vi "sendNoAckToClient.vi"(8 "error in (no error)":errorcluster, 10 "tcpPacket":string, 11 "tcpServerCmd in":refnum<class "TcpServerCmd.lvclass">) -> (0 "error out":errorcluster, 2 "tcpPacket":string, 3 "tcpServerCmd out":refnum<class "TcpServerCmd.lvclass">)   [LabVIEW 2018, in "TcpServerCmd.lvclass"]
doc: "Send the noAck to the TCP Client."
uses:
  TcpServerCmd.lvclass
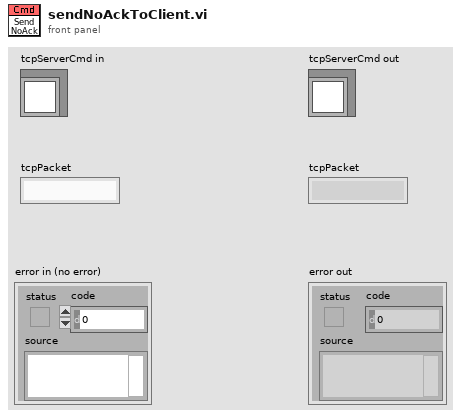
[diagram p1: front panel]
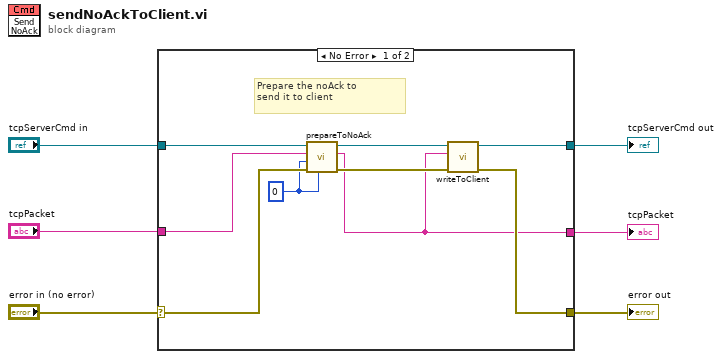
[diagram p0: block diagram]
diagram:
  n1 = case shown="No Error" "error in (no error)" {
    selector: "error in (no error)" -> [w11 w18]
    tunnel: [w14 w18] -> w5
    tunnel: [w15 w17] -> w3
    tunnel: "tcpServerCmd in" -> [w13 w17]
    tunnel: "tcpPacket" -> [w8 w16]
    tunnel: [w7 w16] -> w1
    frame No Error {
      w9 = 0 ("lostCmdId")
      # "Prepare the noAck to\nsend it to client"
      n2 = call "prepareToNoAck.vi"("iteration"=w9, "error in (no error)"=w11, "lostCmdId"=w9, "cmd"=w8, "tcpServerCmd in"=w13) -> ("error out"=w10:errorcluster, "JSON string"=w7:string, "tcpServerCmd out"=w12:refnum<class "TcpServerCmd.lvclass">)  [unwired: 4 in]
      n3 = call "writeToClient.vi"("error in (no error)"=w10, "packet"=w7, "tcpServerCmd in"=w12) -> ("error out"=w14:errorcluster, "tcpServerCmd out"=w15:refnum<class "TcpServerCmd.lvclass">)  [unwired: 7 in]
    }
    frame Error {
    }
  }
  "error out" <- w5
  "tcpServerCmd out" <- w3
  "tcpPacket" <- w1
